vi "Handle Command.vi"(5 "Preceding Items":refnum<class "Item.lvclass">[](array[class]), 7 "Command":string, 8 "error in (no error)":errorcluster, 9 "Active Build Configuration":string, 10 "Selected Items":string[][](array[string]), 11 "ZIP Item in":refnum<class "ZIP Item.lvclass">) -> (0 "error out":errorcluster, 1 "Steps to Build":refnum<class "Build Step.lvclass">[](array[class]), 2 "LV Documents to Open":path[](array[path]), 3 "ZIP Item out":refnum<class "ZIP Item.lvclass">)   [LabVIEW 2019, in "ZIP.lvlib" / "ZIP Item.lvclass"]
uses:
  ZIP Item.lvclass
  libs/Solution.lvlibp/Solution/Item/Item.lvclass
  libs/Solution.lvlibp/Solution/Build Item/Build Step.lvclass
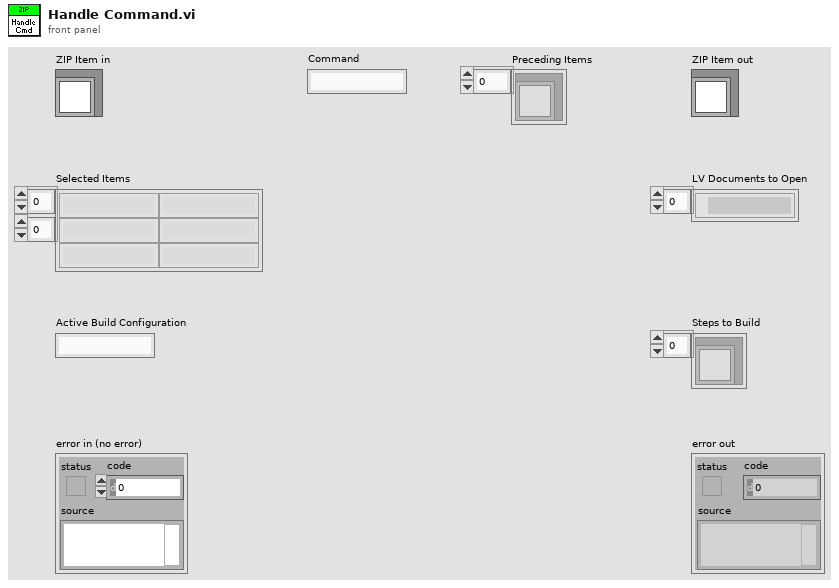
[diagram p1: front panel]
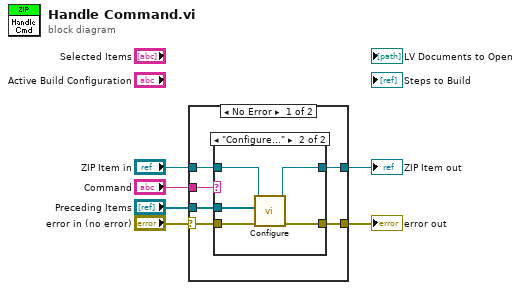
[diagram p0: block diagram]
diagram:
  n1 = case shown="No Error" "error in (no error)" {
    selector: "error in (no error)" -> [w12 w20]
    tunnel: [w11 w20] -> w5
    tunnel: "ZIP Item in" -> [w10 w21]
    tunnel: [w9 w21] -> w3
    tunnel: "Preceding Items" -> [w8 _]
    tunnel: "Command" -> [w7 _]
    frame No Error {
      n2 = case shown="\"Configure...\"" w7 {
        tunnel: w12 -> [w13 w19]
        tunnel: [w13 w18] -> w11
        tunnel: w10 -> [w14 w17]
        tunnel: [w14 w16] -> w9
        tunnel: w8 -> [_ w15]
        frame Default {
        }
        frame "Configure..." {
          n3 = call "Configure.vi"("error in (no error)"=w19, "Preceding Items"=w15, "ZIP Item in"=w17) -> ("error out"=w18:errorcluster, "ZIP Item out"=w16:refnum<class "ZIP Item.lvclass">)  [unwired: 7 in]
        }
      }
    }
    frame Error {
    }
  }
  "error out" <- w5
  "ZIP Item out" <- w3
